vi "get peak height.vi"(9 "Waveform Graph":dbl[][](array[numeric]), 11 "y":dbl=211.0) -> (1 "Array":dbl[](array[numeric]), 3 "mean":dbl format="%0.4f", 4 "mean 2":dbl format="%0.2f", 5 "s? t:f":dbl)   [LabVIEW 2016]
uses:
  <vilib>/Analysis/baseanly.llb/Mean (DBL).vi
  <vilib>/Analysis/NI_AALBase.lvlib
panel:
  out "x/y 3":dbl
  out "x/y 2":dbl
  out "sum 3":dbl
  out "sum 2":dbl
  out "sum":dbl
  out "x/y":dbl
  out "Waveform Graph 4":dbl[](graph)
  out "Waveform Graph 3":dbl[](graph)
  out "Waveform Graph 2":dbl[](graph)
  out "max value":dbl
  out "max index(es)":i32
  out "percent level settings":T1={"method"=enum."auto select", "histogram size"=256, "histogram method"=enum."mode", "reserved"=1.0} {"reserved" format="%0.2f"}
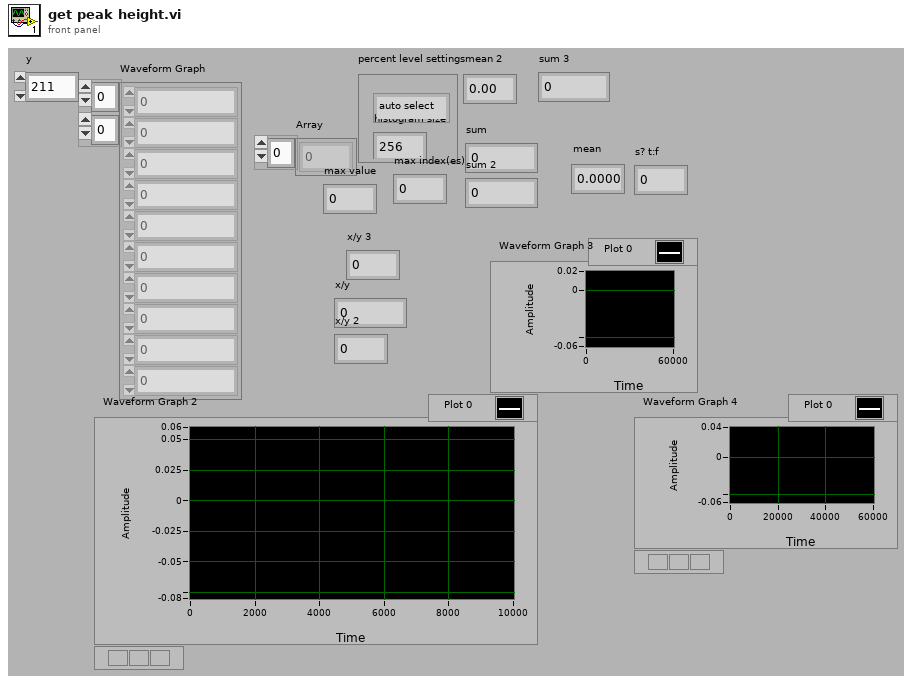
[diagram p1: front panel]
types:
  T1 = cluster{"method":enum32{"histogram", "peak", "auto select"}, "histogram size":i32, "histogram method":enum16{"mode"}, "reserved":dbl}
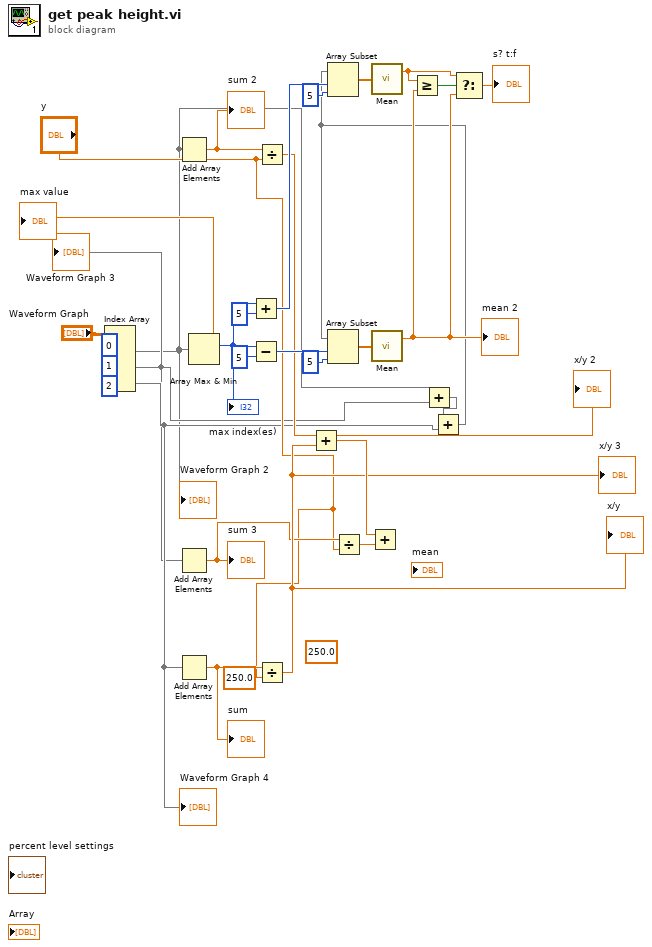
[diagram p0: block diagram]
diagram:
  (unwired) 250.0 ("y")
  (unwired) 250.0 ("y")
  n1 = Index Array(array="Waveform Graph", index (row) #1=0 ("index (row)"), index (row) #2=1 ("disabled index (col)"), index (row) #3=2 ("disabled index (row)")) -> (element #1=w3:dbl[], element #2=w6:dbl[], element #3=w7:dbl[])  [unwired: 3 in]
  "Waveform Graph 2" <- w3
  "Waveform Graph 3" <- w6
  "Waveform Graph 4" <- w7
  n2 = Add Array Elements(numeric array=w3) -> (sum=w14:dbl)
  "sum 2" <- w14
  n3 = Add Array Elements(numeric array=w6) -> (sum=w11:dbl)
  "sum 3" <- w11
  n4 = Add Array Elements(numeric array=w7) -> (sum=w9:dbl)
  "sum" <- w9
  n5 = Array Max & Min(array=w3) -> (max value=→"max value":dbl, max index (indices)=w15:i32)  [unwired: 2 out]
  "max index(es)" <- w15
  n6 = Add(x=w15, y=5) -> (x+y=w30:i32)
  n7 = Subtract(x=w15, y=5) -> (x-y=w25:i32)
  n8 = Divide(x=w14, y="y") -> (x/y=w13:dbl)
  "x/y 2" <- w13
  n9 = Divide(x=w9, y="y") -> (x/y=w12:dbl)
  "x/y" <- w12
  "x/y 3" <- w12
  n10 = Add(x=w13, y=w12) -> (x+y=w16:dbl)
  n11 = Divide(x=w11, y="y") -> (x/y=w10:dbl)
  n12 = Add(x=w16, y=w10) -> ()  [unwired: 1 out]
  n13 = Add(x=w3, y=w6) -> (x+y=w5:dbl[])
  n14 = Add(x=w5, y=w7) -> (x+y=w2:dbl[])
  n15 = Array Subset(array=w2, index=w30, length=5) -> (w28:dbl[])
  n16 = Array Subset(array=w2, index=w25, length=5) -> (w1:dbl[])
  n17 = call-poly <vilib>:"Mean.vi"("X"=w28) -> ("mean"=w23:dbl)  [unwired: 1 out]
  n18 = call-poly <vilib>:"Mean.vi"("X"=w1) -> ("mean"=w22:dbl)  [unwired: 1 out]
  "mean 2" <- w22
  n19 = Greater Or Equal?(x=w23, y=w22) -> (x >= y?=w24:bool)
  n20 = Select(t=w23, s=w24, f=w22) -> (s? t:f=→"s? t:f":dbl)
